vi "DHE_ImtypeActions.vi"(8 "error in (no error)":errorcluster, 10 "imtype":string, 11 "fd in":i32) -> (0 "error out":errorcluster, 3 "fd out":i32)   [LabVIEW 2016]
uses:
  DBSHAND/private/vis/DatabaseHand_Element_Get(bool).vi
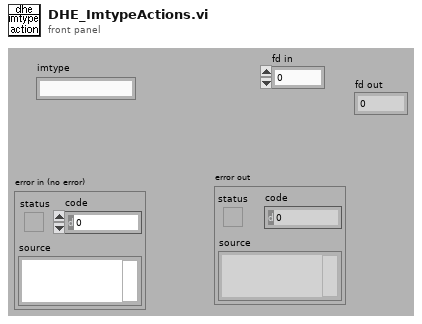
[diagram p1: front panel]
types:
  T1 = typedef "DatabaseHand_RefNum.ctl" = refnum<vi>
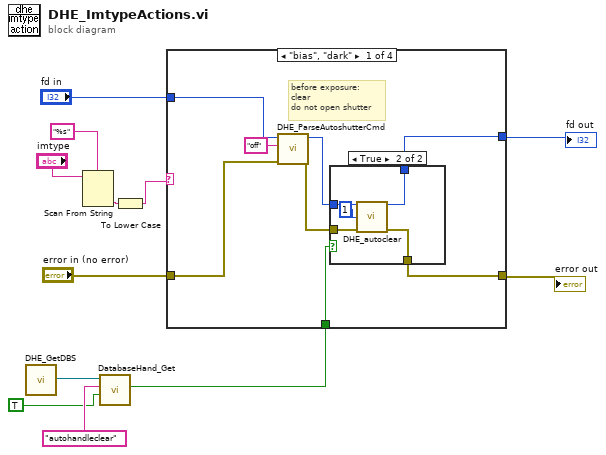
[diagram p0: block diagram]
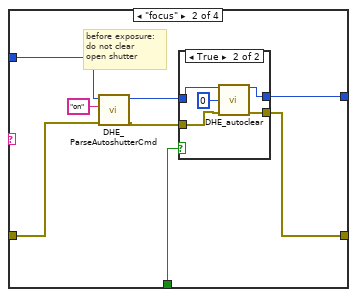
[diagram p3: hidden frame]
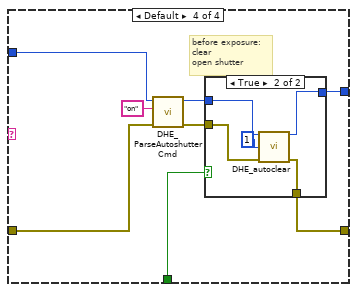
[diagram p6: hidden frame]
diagram:
  n1 = call "DHE_GetDBS.vi"() -> ("DHE_DBSRef"=w4:T1)  [unwired: 9 out]
  n2 = Scan From String(format string="%s", input string="imtype") -> (output 1=w10:string)  [unwired: 2 in, 4 out]
  n3 = call-poly "DatabaseHand_Get.vi"("default value"=TRUE, "name"="autohandleclear", "Database RefNum in"=w4) -> ("value"=w1:bool)  [unwired: 2 in, 6 out]
  n4 = To Lower Case(string=w10) -> (all lower case string=w9:string)
  n5 = case shown="\"bias\", \"dark\"" w9 {
    tunnel: "error in (no error)" -> [w18 w32 w43 w50]
    tunnel: [w17 w34 w43 w48] -> w7
    tunnel: "fd in" -> [w20 w29 w44 w51]
    tunnel: [w14 w35 w44 w46] -> w5
    tunnel: w1 -> [w13 w28 _ w45]
    frame "bias", "dark" {
      # "before exposure:\nclear\ndo not open shutter"
      n6 = call "DHE_ParseAutoshutterCmd.vi"("error in (no error)"=w18, "argument"="off", "fd"=w20) -> ("error out"=w16:errorcluster, "fd out"=w15:i32)  [unwired: 7 out]
      n7 = case shown="True" w13 {
        tunnel: [w21 w26] -> w17
        tunnel: w16 -> [w21 w25]
        tunnel: w15 -> [w22 w24]
        tunnel: [w22 w23] -> w14
        frame False {
        }
        frame True {
          n8 = call "DHE_autoclear.vi"("fd"=w24, "flag"=i16 1, "error in (no error)"=w25) -> ("fd out"=w23:i32, "error out"=w26:errorcluster)  [unwired: 11 out]
        }
      }
    }
    frame "focus" {
      # "before exposure:\ndo not clear\nopen shutter"
      n9 = call "DHE_ParseAutoshutterCmd.vi"("error in (no error)"=w32, "argument"="on", "fd"=w29) -> ("error out"=w31:errorcluster, "fd out"=w30:i32)  [unwired: 7 out]
      n10 = case shown="True" w28 {
        tunnel: [w37 w42] -> w35
        tunnel: [w36 w41] -> w34
        tunnel: w31 -> [w36 w39]
        tunnel: w30 -> [w37 w38]
        frame False {
        }
        frame True {
          n11 = call "DHE_autoclear.vi"("fd"=w38, "flag"=i16 0, "error in (no error)"=w39) -> ("fd out"=w42:i32, "error out"=w41:errorcluster)  [unwired: 11 out]
        }
      }
    }
    frame "none" {
      # "leave it alone"
    }
    frame Default {
      # "before exposure:\nclear\nopen shutter"
      n12 = call "DHE_ParseAutoshutterCmd.vi"("error in (no error)"=w50, "argument"="on", "fd"=w51) -> ("error out"=w49:errorcluster, "fd out"=w47:i32)  [unwired: 7 out]
      n13 = case shown="True" w45 {
        tunnel: w49 -> [w54 w59]
        tunnel: [w54 w58] -> w48
        tunnel: w47 -> [w53 w57]
        tunnel: [w53 w55] -> w46
        frame False {
        }
        frame True {
          n14 = call "DHE_autoclear.vi"("fd"=w57, "flag"=i16 1, "error in (no error)"=w59) -> ("fd out"=w55:i32, "error out"=w58:errorcluster)  [unwired: 11 out]
        }
      }
    }
  }
  "error out" <- w7
  "fd out" <- w5
